vi "writeread(sub).vi"(0 "delay before read (ms)":u32=500, 1 "resourcein":refnum<visa-resource-name>, 2 "New Value":dbl caption="s", 3 "Command":dbl, 4 "errorin":errorcluster) -> (5 "resourceout":refnum<visa-resource-name>, 6 "readstring":string, 7 "errorout":errorcluster)   [LabVIEW 2015]
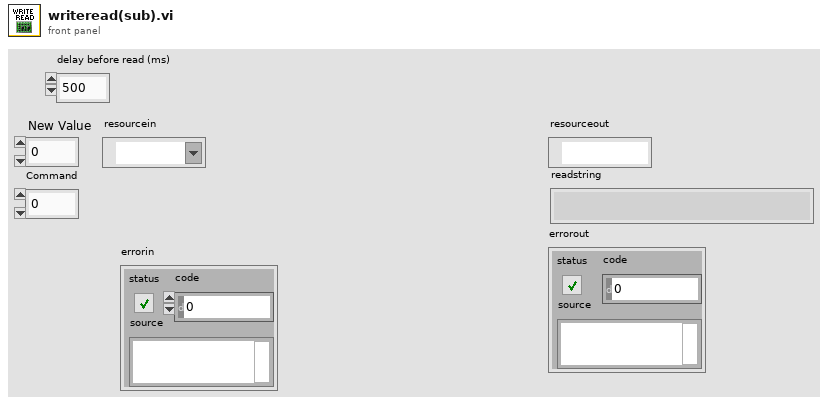
[diagram p1: front panel]
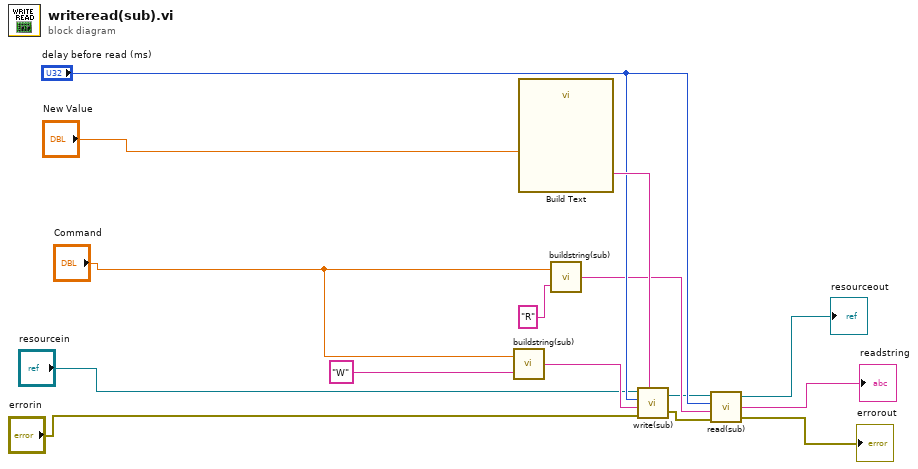
[diagram p0: block diagram]
diagram:
  n1 = call "buildstring(sub).vi"("Prefix"="W", "Command"="Command") -> ("Commandstring"=w14:string)
  n2 = call "Build Text"("s"="New Value") -> ("Result"=w13:string)  [unwired: 13 in, 1 out]
  n3 = call "buildstring(sub).vi"("Prefix"="R", "Command"="Command") -> ("Commandstring"=w10:string)
  n4 = call "write(sub).vi"("resourcein"="resourcein", "readdelay"="delay before read (ms)", "writestring"=w14, "errorin"="errorin", "payload"=w13) -> ("resourceout"=w9:refnum<visa-resource-name>, "errorout"=w12:errorcluster)
  n5 = call "read(sub).vi"("errorin"=w12, "writestring"=w10, "readdelay"="delay before read (ms)", "resourcein"=w9) -> ("errorout"=→"errorout":errorcluster, "readstring"=→"readstring":string, "resourceout"=→"resourceout":refnum<visa-resource-name>)
